vi "parse_Flatearth.vi"(0 "Parent path":path) -> (4 "FlatEarth Inputs":T1)   [LabVIEW 2015]
uses:
  FlatEarth Inputs.ctl
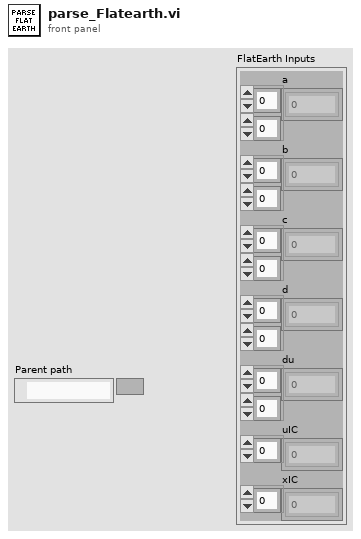
[diagram p1: front panel]
types:
  T1 = typedef "FlatEarth Inputs.ctl" = cluster{"a":dbl[][], "b":dbl[][], "c":dbl[][], "d":dbl[][], "du":dbl[][], "uIC":dbl[], "xIC":dbl[]}
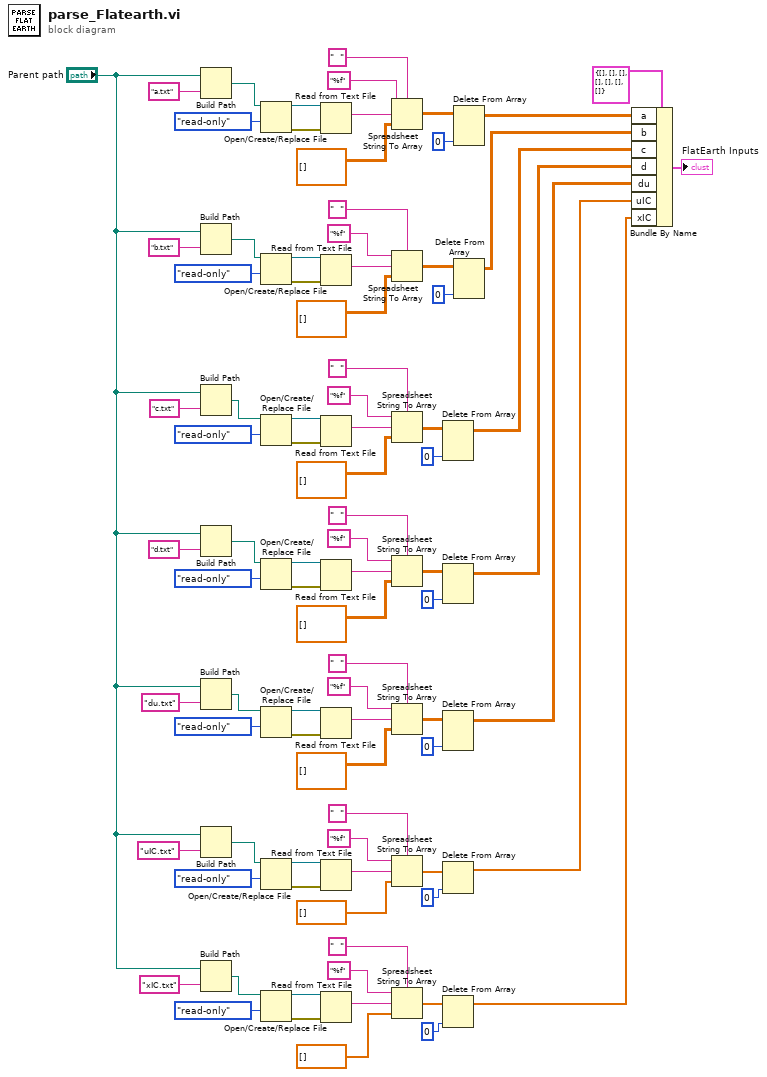
[diagram p0: block diagram]
diagram:
  n1 = Build Path(base path="Parent path", name or relative path="a.txt") -> (appended path=w44:path)
  n2 = Build Path(base path="Parent path", name or relative path="b.txt") -> (appended path=w42:path)
  n3 = Build Path(base path="Parent path", name or relative path="c.txt") -> (appended path=w40:path)
  n4 = Build Path(base path="Parent path", name or relative path="d.txt") -> (appended path=w38:path)
  n5 = Build Path(base path="Parent path", name or relative path="du.txt") -> (appended path=w36:path)
  n6 = Build Path(base path="Parent path", name or relative path="uIC.txt") -> (appended path=w34:path)
  n7 = Build Path(base path="Parent path", name or relative path="xIC.txt") -> (appended path=w32:path)
  n8 = Open/Create/Replace File(file path (use dialog)=w44, access (0:read/write)=enum16{"read/write", "read-only", "write-only"}."read-only") -> (refnum out=w85:refnum<file>, error out=w86:errorcluster)  [unwired: 4 in, 1 out]
  n9 = Open/Create/Replace File(file path (use dialog)=w42, access (0:read/write)=enum16{"read/write", "read-only", "write-only"}."read-only") -> (refnum out=w78:refnum<file>, error out=w77:errorcluster)  [unwired: 4 in, 1 out]
  n10 = Open/Create/Replace File(file path (use dialog)=w40, access (0:read/write)=enum16{"read/write", "read-only", "write-only"}."read-only") -> (refnum out=w73:refnum<file>, error out=w74:errorcluster)  [unwired: 4 in, 1 out]
  n11 = Open/Create/Replace File(file path (use dialog)=w38, access (0:read/write)=enum16{"read/write", "read-only", "write-only"}."read-only") -> (refnum out=w66:refnum<file>, error out=w65:errorcluster)  [unwired: 4 in, 1 out]
  n12 = Open/Create/Replace File(file path (use dialog)=w36, access (0:read/write)=enum16{"read/write", "read-only", "write-only"}."read-only") -> (refnum out=w61:refnum<file>, error out=w62:errorcluster)  [unwired: 4 in, 1 out]
  n13 = Open/Create/Replace File(file path (use dialog)=w34, access (0:read/write)=enum16{"read/write", "read-only", "write-only"}."read-only") -> (refnum out=w49:refnum<file>, error out=w50:errorcluster)  [unwired: 4 in, 1 out]
  n14 = Open/Create/Replace File(file path (use dialog)=w32, access (0:read/write)=enum16{"read/write", "read-only", "write-only"}."read-only") -> (refnum out=w55:refnum<file>, error out=w56:errorcluster)  [unwired: 4 in, 1 out]
  n15 = Read from Text File(file (use dialog)=w85, error in=w86) -> (text=w84:string)  [unwired: 2 in, 3 out]
  n16 = Read from Text File(file (use dialog)=w78, error in=w77) -> (text=w79:string)  [unwired: 2 in, 3 out]
  n17 = Read from Text File(file (use dialog)=w73, error in=w74) -> (text=w72:string)  [unwired: 2 in, 3 out]
  n18 = Read from Text File(file (use dialog)=w66, error in=w65) -> (text=w67:string)  [unwired: 2 in, 3 out]
  n19 = Read from Text File(file (use dialog)=w61, error in=w62) -> (text=w60:string)  [unwired: 2 in, 3 out]
  n20 = Read from Text File(file (use dialog)=w49, error in=w50) -> (text=w48:string)  [unwired: 2 in, 3 out]
  n21 = Read from Text File(file (use dialog)=w55, error in=w56) -> (text=w54:string)  [unwired: 2 in, 3 out]
  n22 = Spreadsheet String To Array(delimiter (Tab)="  ", format string="%f", spreadsheet string=w84, array type (2D Dbl)=dbl[][] []) -> (array=w23:dbl[][])
  n23 = Spreadsheet String To Array(delimiter (Tab)="  ", format string="%f", spreadsheet string=w79, array type (2D Dbl)=dbl[][] []) -> (array=w21:dbl[][])
  n24 = Spreadsheet String To Array(delimiter (Tab)="  ", format string="%f", spreadsheet string=w72, array type (2D Dbl)=dbl[][] []) -> (array=w19:dbl[][])
  n25 = Spreadsheet String To Array(delimiter (Tab)="  ", format string="%f", spreadsheet string=w67, array type (2D Dbl)=dbl[][] []) -> (array=w17:dbl[][])
  n26 = Spreadsheet String To Array(delimiter (Tab)="  ", format string="%f", spreadsheet string=w60, array type (2D Dbl)=dbl[][] []) -> (array=w15:dbl[][])
  n27 = Spreadsheet String To Array(delimiter (Tab)="  ", format string="%f", spreadsheet string=w48, array type (2D Dbl)=dbl[] []) -> (array=w14:dbl[])
  n28 = Spreadsheet String To Array(delimiter (Tab)="  ", format string="%f", spreadsheet string=w54, array type (2D Dbl)=dbl[] []) -> (array=w11:dbl[])
  n29 = Delete From Array(array=w19, index (col)=0 ("disabled index (col)")) -> (array with subset deleted=w3:dbl[][])  [unwired: 2 in, 1 out]
  n30 = Delete From Array(array=w17, index (col)=0 ("disabled index (col)")) -> (array with subset deleted=w4:dbl[][])  [unwired: 2 in, 1 out]
  n31 = Delete From Array(array=w15, index (col)=0 ("disabled index (col)")) -> (array with subset deleted=w5:dbl[][])  [unwired: 2 in, 1 out]
  n32 = Delete From Array(array=w14, index=0 ("disabled index (col)")) -> (array with subset deleted=w6:dbl[])  [unwired: 1 in, 1 out]
  n33 = Delete From Array(array=w11, index=0 ("disabled index (col)")) -> (array with subset deleted=w7:dbl[])  [unwired: 1 in, 1 out]
  n34 = Delete From Array(array=w23, index (col)=0 ("disabled index (col)")) -> (array with subset deleted=w8:dbl[][])  [unwired: 2 in, 1 out]
  n35 = Delete From Array(array=w21, index (col)=0 ("disabled index (col)")) -> (array with subset deleted=w2:dbl[][])  [unwired: 2 in, 1 out]
  n36 = Bundle By Name(cluster=T1 {"a"=[], "b"=[], "c"=[], "d"=[], "du"=[], "uIC"=[], "xIC"=[]}, "a"=w8, "b"=w2, "c"=w3, "d"=w4, "du"=w5, "uIC"=w6, "xIC"=w7) -> (→"FlatEarth Inputs":T1)
